vi "Phasor Compute Phasor from Decay v2.vi"(8 "Error In":errorcluster, 9 "Phasor Frequency":dbl[unit], 11 "Time-Gated Decay":cluster{"t Array":dbl[], "I Array":dbl[]}) -> (0 "Error Out":errorcluster, 1 "z":cdb, 2 "s":dbl, 3 "g":dbl, 5 "Total Intensity":dbl)   [LabVIEW 2021, in "Phasor.lvlib"]
doc: "Computes the discrete phasor of the provided decay, assuming that the time array has ns unit.\n\nThe trigonometric functions are evaluated the first time a new time array is provided, and saved for subseqeunt calls with the same time array."
uses:
  Phasor.lvlib
  66495d7f-c188-42fb-9dc1-6117c0cf50cd.vi
  bd8958be-9d91-49e3-98a2-14b3b9abff81.vi
  Math/ix/ix [DBL].vi
  <vilib>/Utility/error.llb/Error Cluster From Error Code.vi
  <vilib>/ErrorRing/Error Ring.xnode
  Math/Math.lvlib
panel:
  # "see the License on the block diagram (Ctrl+E or Window:Show Block Diagram)"
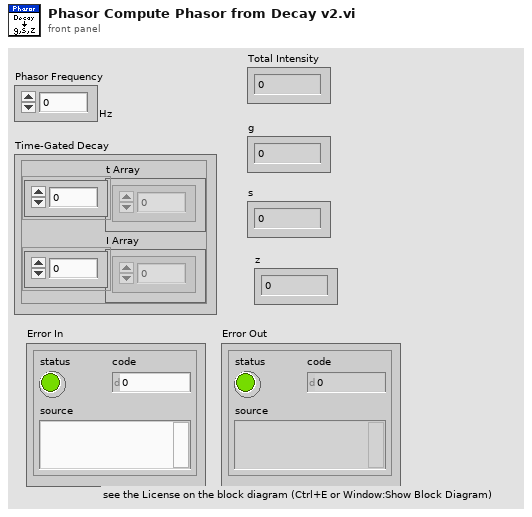
[diagram p1: front panel]
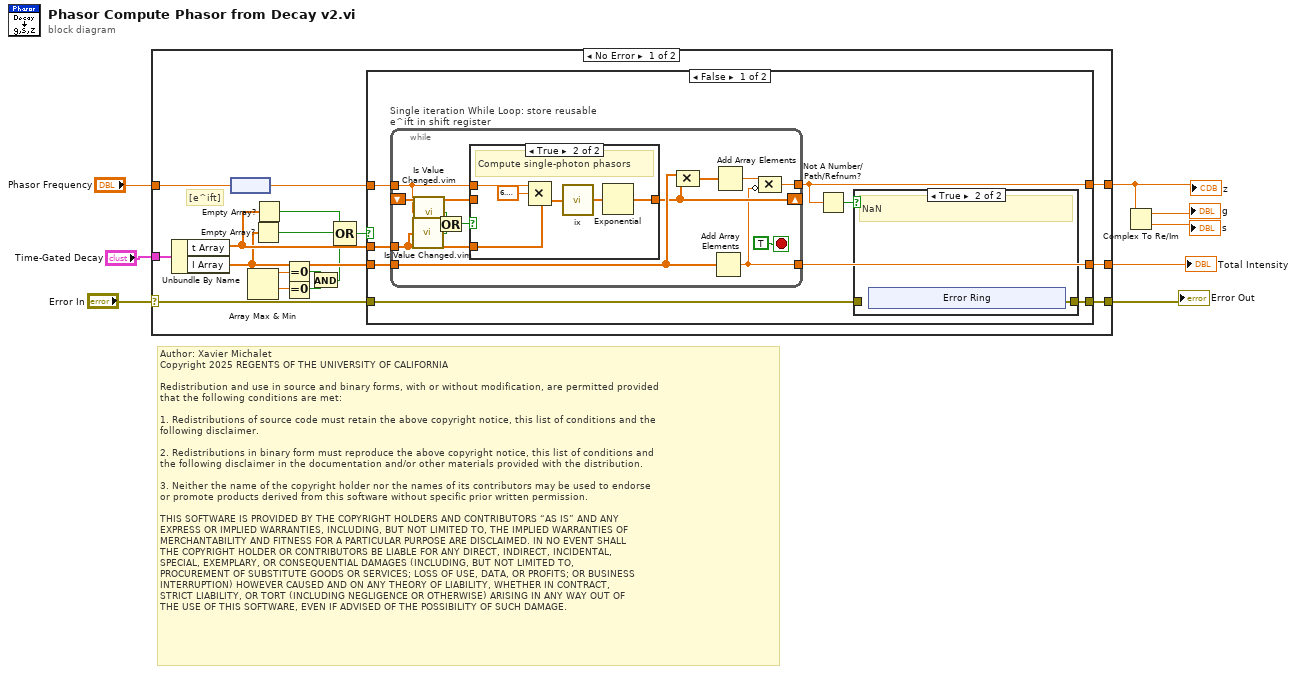
[diagram p0: block diagram]
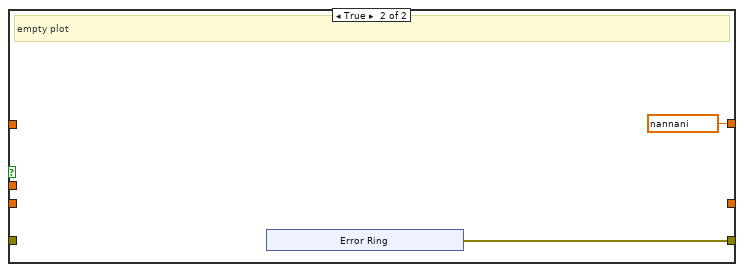
[diagram p4: hidden frame]
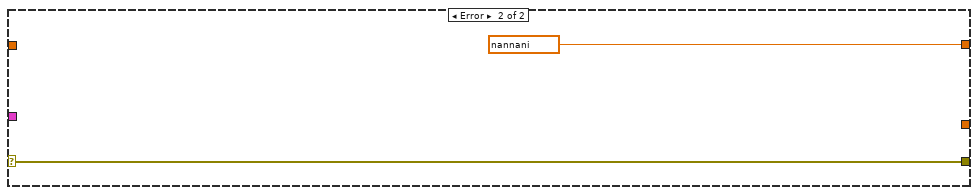
[diagram p5: hidden frame]
diagram:
  # "Author: Xavier Michalet\nCopyright 2025 REGENTS OF THE UNIVERSITY OF CALIFORNIA\n\nRedistribution and use in source and binary forms, with or without modification, are permitted provided\nthat the following conditions are met:\n\n1. Redistributions of source code must retain the above copyright notice, this list of conditions and the\nfollowing disclaimer.\n\n2. Redistributions in binary form must reproduce the above copyright notice, this list of conditions and\nthe following disclaimer in the documentation and/or other materials provided with the distribution.\n\n3. Neither the name of the copyright holder nor the names of its contributors may be used to endorse \nor promote products derived from this software without specific prior written permission.\n\nTHIS SOFTWARE IS PROVIDED BY THE COPYRIGHT HOLDERS AND CONTRIBUTORS “AS IS” AND ANY \nEXPRESS OR IMPLIED WARRANTIES, INCLUDING, BUT NOT LIMITED TO, THE IMPLIED WARRANTIES OF\nMERCHANTABILITY AND FITNESS FOR A PARTICULAR PURPOSE ARE DISCLAIMED. IN NO EVENT SHALL\nTHE COPYRIGHT HOLDER OR CONTRIBUTORS BE LIABLE FOR ANY DIRECT, INDIRECT, INCIDENTAL, \nSPECIAL, EXEMPLARY, OR CONSEQUENTIAL DAMAGES (INCLUDING, BUT NOT LIMITED TO, \nPROCUREMENT OF SUBSTITUTE GOODS OR SERVICES; LOSS OF USE, DATA, OR PROFITS; OR BUSINESS\nINTERRUPTION) HOWEVER CAUSED AND ON ANY THEORY OF LIABILITY, WHETHER IN CONTRACT, \nSTRICT LIABILITY, OR TORT (INCLUDING NEGLIGENCE OR OTHERWISE) ARISING IN ANY WAY OUT OF\nTHE USE OF THIS SOFTWARE, EVEN IF ADVISED OF THE POSSIBILITY OF SUCH DAMAGE."
  n1 = case shown="No Error" "Error In" {
    selector: "Error In" -> [w17 w66]
    tunnel: "Phasor Frequency" -> [w25 _]
    tunnel: [w24 cdb nan+nani] -> w4
    tunnel: "Time-Gated Decay" -> [w23 _]
    tunnel: [w18 w66] -> w5
    tunnel: [w9 _] -> w1
    frame No Error {
      # "[e^ift]"
      n2 = Unbundle By Name(w23) -> ("t Array"=w22:dbl[], "I Array"=w15:dbl[])
      n3 = node(w25) -> (w16:dbl)
      n4 = Array Max & Min(array=w15) -> (max value=w14:dbl, min value=w13:dbl)  [unwired: 2 out]
      n5 = Empty Array?(array=w15) -> (empty?=w20:bool)
      n6 = Empty Array?(array=w22) -> (empty?=w21:bool)
      n7 = Equal To 0?(x=w14) -> (x = 0?=w12:bool)
      n8 = Equal To 0?(x=w13) -> (x = 0?=w11:bool)
      n9 = And(x=w12, y=w11) -> (x .and. y?=w10:bool)
      n10 = Compound Arithmetic op=OR(w21, w20, w10) -> (w19:bool)
      n11 = case shown="False" w19 {
        tunnel: w16 -> [w33 _]
        tunnel: [w30 cdb nan+nani] -> w24
        tunnel: w22 -> [w32 _]
        tunnel: w15 -> [w31 _]
        tunnel: [w28 w61] -> w18
        tunnel: w17 -> [w29 _]
        tunnel: [w26 _] -> w9
        frame False {
          n12 = while "Single iteration While Loop: store reusable e^ift in shift register" {
            tunnel: w33 -> [w44]
            tunnel: w32 -> [w41]
            tunnel: w31 -> [w47]
            tunnel: [w52] -> w30
            shift-right: [w46] -> _
            shift-left: _ -> [w48]
            tunnel: [w40] -> w26
            stop <- TRUE stop-if-true
            n13 = call "Is Value Changed.vim"("value"=w41) -> ("changed or first call?"=w42:bool)
            n14 = call "Is Value Changed.vim"("value"=w44) -> ("changed or first call?"=w43:bool)
            n15 = Or(x=w43, y=w42) -> (x .or. y?=w49:bool)
            n16 = case shown="True" w49 {
              tunnel: [w53 w54] -> w46
              tunnel: w41 -> [_ w55]
              tunnel: w44 -> [_ w58]
              tunnel: w48 -> [w53 _]
              frame False {
                # "no need to recompute"
              }
              frame True {
                # "Compute single-photon phasors"
                n17 = Compound Arithmetic op=MULTIPLY(w58, 6.283185307179586, w55) -> (w57:dbl[])
                n18 = call-poly "ix.vi"("x (1)"=w57) -> ("i.(x)"=w56:cdb[])
                n19 = Exponential(1:w56) -> (0:w54:cdb[])
              }
            }
            n20 = Compound Arithmetic op=MULTIPLY(w47, w46) -> (w50:cdb[])
            n21 = Add Array Elements(numeric array=w47) -> (sum=w40:dbl)
            n22 = Add Array Elements(numeric array=w50) -> (sum=w51:cdb)
            n23 = Compound Arithmetic op=MULTIPLY(w51, invert w40) -> (w52:cdb)
          }
          n24 = Not A Number/Path/Refnum?(number/path/refnum=w30) -> (NaN/Path/Refnum?=w27:bool)
          n25 = case shown="True" w27 {
            tunnel: w29 -> [w34 _]
            tunnel: [w34 w35] -> w28
            frame False {
            }
            frame True {
              # "NaN"
              n26 = xnode "Error Ring"() -> ("error out"=w35:errorcluster)
            }
          }
        }
        frame True {
          # "empty plot"
          n27 = xnode "Error Ring"() -> ("error out"=w61:errorcluster)
        }
      }
    }
    frame Error {
    }
  }
  "Error Out" <- w5
  "z" <- w4
  "Total Intensity" <- w1
  n28 = Complex To Re/Im(x + iy=w4) -> (x=→"g":dbl, y=→"s":dbl)
